vi "UI_Initialize.vi"(8 "error in (no error)":errorcluster, 11 "Module in":refnum<class "Module.lvclass">) -> (0 "error out":errorcluster, 3 "Module out":refnum<class "Module.lvclass">)   [LabVIEW 2025, in "Module.lvlib" / "Module.lvclass"]
uses:
  Module.lvclass
  <vilib>/Test Bench Framework/Client Message(Context).vi
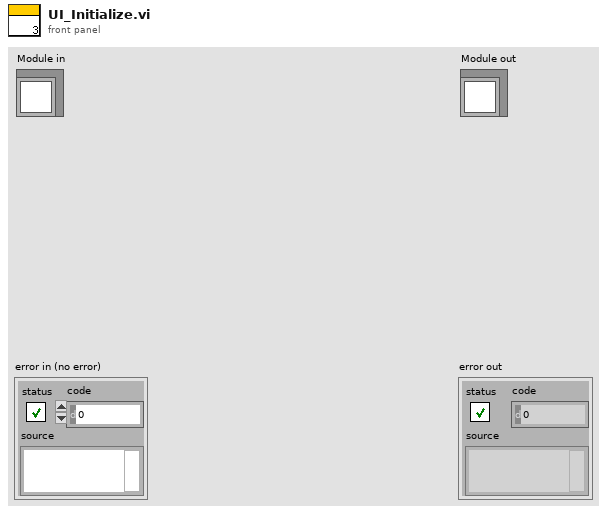
[diagram p1: front panel]
types:
  T1 = cluster{"ModelName":string, "This VI":refnum<vi>}
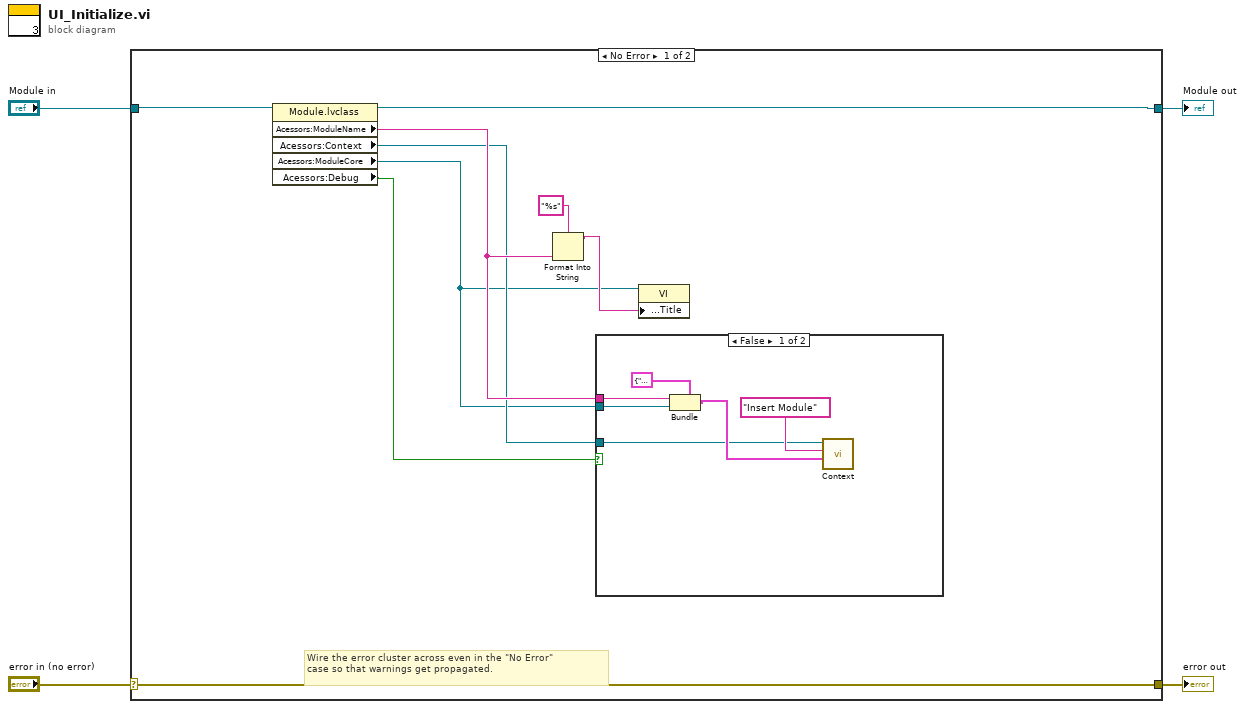
[diagram p0: block diagram]
diagram:
  n1 = case shown="No Error" "error in (no error)" {
    selector: "error in (no error)" -> [w13 w21]
    tunnel: [w13 w21] -> w3
    tunnel: [w7 w20] -> w1
    tunnel: "Module in" -> [w8 w20]
    frame No Error {
      # "Wire the error cluster across even in the \"No Error\"\ncase so that warnings get propagated."
      n2 = property class="Module.lvclass"(reference=w8) -> (reference out=w7:refnum<class "Module.lvclass">, "Acessors:ModuleName"=w10:string, "Acessors:Context"=w9:refnum<vi>, "Acessors:ModuleCore"=w6:refnum<vi>, "Acessors:Debug"=w5:bool)  [unwired: 1 in, 1 out]
      n3 = Format Into String(format string="%s", w10) -> (resulting string=w11:string)  [unwired: 2 in, 1 out]
      n4 = case shown="False" w5 {
        tunnel: w10 -> [w16 _]
        tunnel: w9 -> [w15 _]
        tunnel: w6 -> [w14 _]
        frame False {
          n5 = Bundle(cluster=T1 {"ModelName"="", "This VI"=refnum}, "ModelName"=w16, "This VI"=w14) -> (w19:T1)
          n6 = call-poly <vilib>:"Context.vi"("Value"=w19, "Msg"="Insert Module", "Context"=w15) -> ()  [unwired: 8 in, 1 out]
        }
        frame True {
        }
      }
      n7 = property class="VI"(reference=w6, "Front Panel.Title"=w11) -> ()  [unwired: 1 in, 2 out]
    }
    frame Error {
    }
  }
  "error out" <- w3
  "Module out" <- w1
